vi "ExTestTemperature.vi"() -> ()   [LabVIEW 2010]
panel:
  out "Current Temperature":dbl format="%.2f"
  out "Thermometer":dbl(slide) min=-150.0 max=0.0 scale format="%.3f"
  in  "Cancel Setting":bool
  out "Temperature Set?":bool
  in  "Temperature":dbl format="%.2f"
  out "error out":errorcluster
  in  "error in (no error)":errorcluster
  # "ExTestTemperature:\nThis example shows how to\nwait for the temperature to \nreach the desired setting.\nNote: not all cameras support\nthe read temperature and a\nfew don't support the setting\nof the temperature."
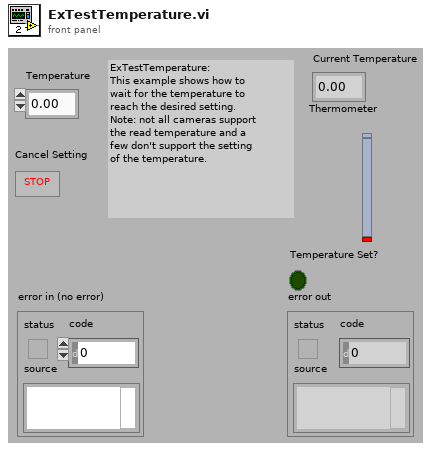
[diagram p1: front panel]
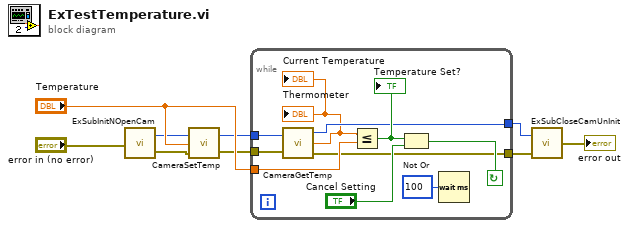
[diagram p0: block diagram]
diagram:
  n1 = call "ExSubInitNOpenCam.vi"("error in (no error)"="error in (no error)") -> ("Camera Handle"=w3:u32, "error out"=w2:errorcluster)
  n2 = call <userlib>:"CameraSetTemp.vi"("error in (no error)"=w2, "Temperature"="Temperature", "Camera Handle"=w3) -> ("error out"=w8:errorcluster, "Camera Handle"=w7:u32)
  n3 = while {
    tunnel: "Temperature" -> [w19]
    tunnel: w8 -> [w15]
    tunnel: w7 -> [w14]
    tunnel: [w13] -> w6
    tunnel: [w12] -> w5
    stop <- w17 continue-if-true
    n4 = call <userlib>:"CameraGetTemp.vi"("Camera Handle"=w14, "error in (no error)"=w15) -> ("Camera Handle"=w13:u32, "Temperature"=w10:dbl, "error out"=w12:errorcluster)
    "Thermometer" <- w10
    "Current Temperature" <- w10
    n5 = Less Or Equal?(x=w10, y=w19) -> (x <= y?=w16:bool)
    "Temperature Set?" <- w16
    n6 = Not Or(1:"Cancel Setting", 2:w16) -> (0:w17:bool)
    n7 = Wait (ms)(milliseconds to wait=u32 100) -> ()  [unwired: 1 out]
  }
  n8 = call "ExSubCloseCamUnInit.vi"("error in (no error)"=w5, "Camera Handle"=w6) -> ("error out"=→"error out":errorcluster)
